vi "TCN.vi"(8 "error in":errorcluster caption="errorIn", 11 "xmlFilePath":path) -> (0 "error out":errorcluster caption="errorOut", 3 "TCN":T1)   [LabVIEW 2017]
uses:
  models/TCN.ctl
  models/Header.ctl
  models/TCN_outputSignal.ctl
  models/TCN_attachedInformation.ctl
  models/TCN_triggerConditions.ctl
  models/TCN_orSignals.ctl
  models/TCN_andSignals.ctl
  models/TCN_pulseClass.ctl
  <vilib>/xml/Load XML File.vi
  <vilib>/xml/NI_XML.lvlib
panel:
  in  "输入簇":T1
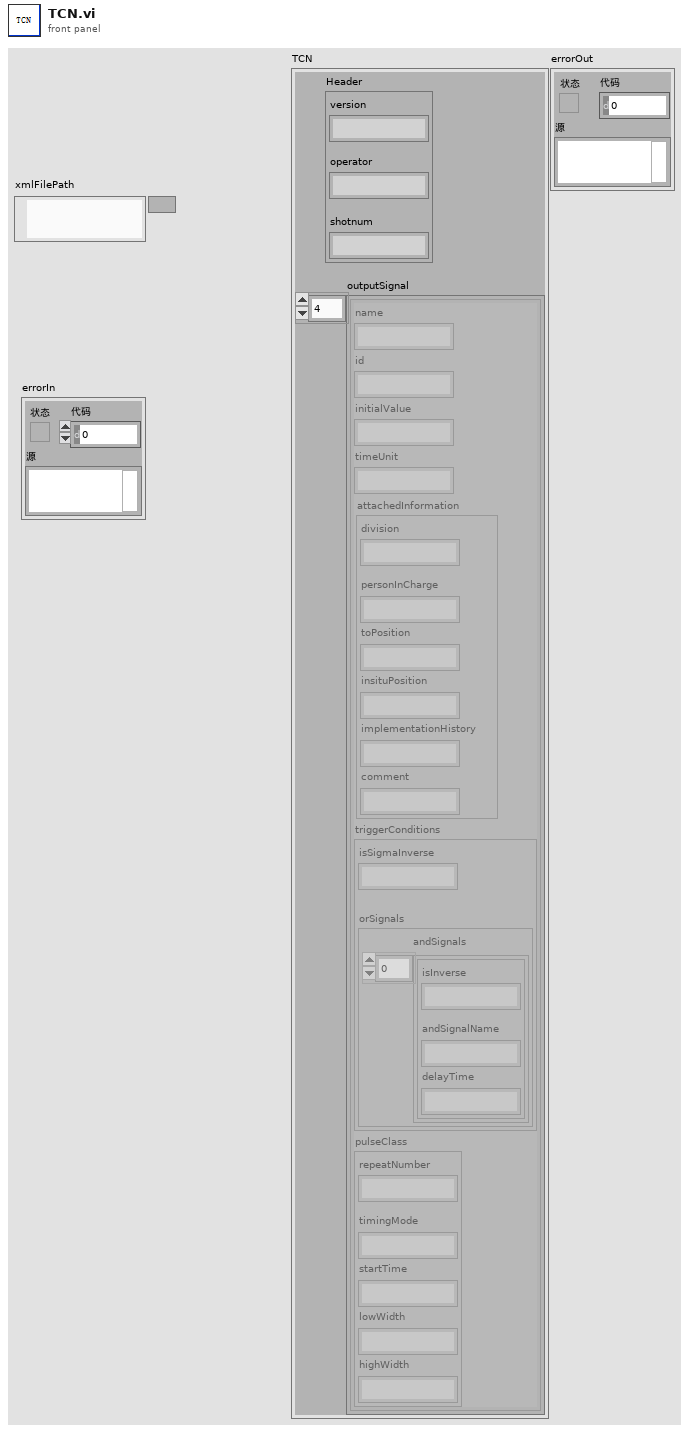
[diagram p1: front panel]
types:
  T1 = typedef "TCN.ctl" = cluster{"Header":T2, "outputSignal":T3[]}
  T2 = typedef "Header.ctl" = cluster{"version":string, "operator":string, "shotnum":string}
  T3 = typedef "TCN_outputSignal.ctl" = cluster{"name":string, "id":string, "initialValue":string, "timeUnit":string, "attachedInformation":T4, "triggerConditions":T5, "pulseClass":T8}
  T4 = typedef "TCN_attachedInformation.ctl" = cluster{"division":string, "personInCharge":string, "toPosition":string, "insituPosition":string, "implementationHistory":string, "comment":string}
  T5 = typedef "TCN_triggerConditions.ctl" = cluster{"isSigmaInverse":string, "orSignals":T6}
  T6 = typedef "TCN_orSignals.ctl" = cluster{"andSignals":T7[]}
  T7 = typedef "TCN_andSignals.ctl" = cluster{"isInverse":string, "andSignalName":string, "delayTime":string}
  T8 = typedef "TCN_pulseClass.ctl" = cluster{"repeatNumber":string, "timingMode":string, "startTime":string, "lowWidth":string, "highWidth":string}
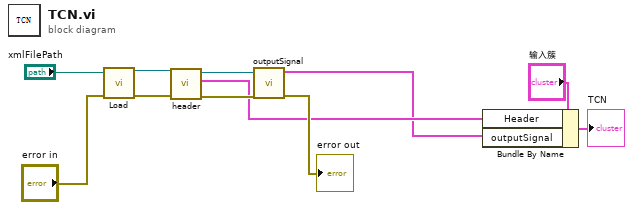
[diagram p0: block diagram]
diagram:
  n1 = call-poly <vilib>:"Load.vi"("path to XML document"="xmlFilePath", "error in (no error)"="error in") -> ("DOM document out"=w9:refnum<k20>, "error out"=w8:errorcluster)  [unwired: 5 in, 7 out]
  n2 = call "header.vi"("errorIn"=w8, "xmlRef"=w9) -> ("errorOut"=w6:errorcluster, "header"=w3:T2, "xmlRef"=w7:refnum<k20>)  [unwired: 7 in]
  n3 = call "outputSignal.vi"("error in"=w6, "xmlRef"=w7) -> ("error out"=→"error out":errorcluster, "outputSignal"=w2:T3[])  [unwired: 8 in]
  n4 = Bundle By Name(cluster="输入簇", "Header"=w3, "outputSignal"=w2) -> (→"TCN":T1)
